vi "Delay.vi"(1 "Stop":bool, 2 "Wait (s)":i32) -> ()   [LabVIEW 2020]
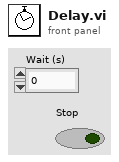
[diagram p1: front panel]
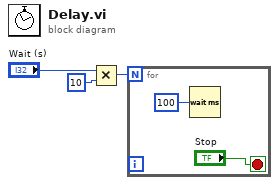
[diagram p0: block diagram]
diagram:
  n1 = Multiply(x="Wait (s)", y=10) -> (x*y=w1:i32)
  n2 = for {
    N: w1 -> [_]
    stop <- "Stop" stop-if-true
    n3 = Wait (ms)(milliseconds to wait=u32 100) -> ()  [unwired: 1 out]
  }
